vi "Write Shield Count.vi"(7 "function":enum16{"Add", "Subtract"}(ring), 8 "error in (no error)":errorcluster, 11 "Shield in":refnum<class "Shield.lvclass">) -> (0 "error out":errorcluster, 3 "Shield out":refnum<class "Shield.lvclass">)   [LabVIEW 2021, in "Shield.lvclass"]
uses:
  Shield.lvclass
  Shield.lvclass/Shield.ctl
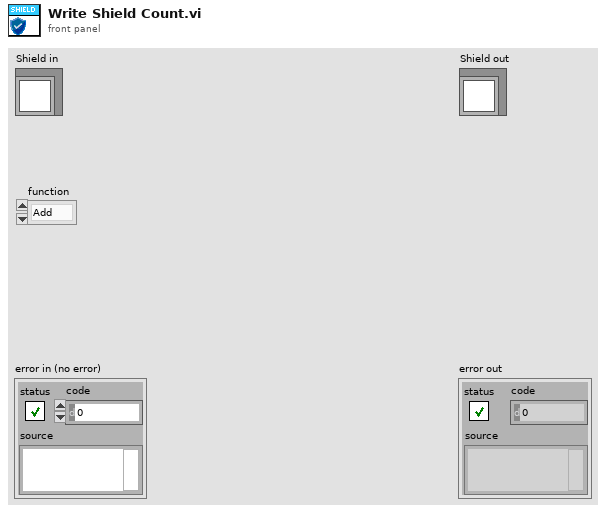
[diagram p1: front panel]
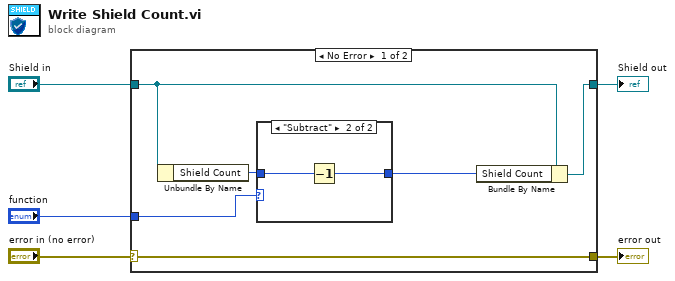
[diagram p0: block diagram]
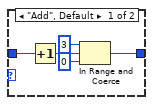
[diagram p2: hidden frame]
diagram:
  n1 = case shown="No Error" "error in (no error)" {
    selector: "error in (no error)" -> [w11 w19]
    tunnel: [w11 w19] -> w4
    tunnel: [w10 w20] -> w2
    tunnel: "Shield in" -> [w7 w20]
    tunnel: "function" -> [w9 _]
    frame No Error {
      n2 = Unbundle By Name(w7) -> ("Shield Count"=w6:u8)
      n3 = case shown="\"Subtract\"" w9 {
        tunnel: w6 -> [w16 w18]
        tunnel: [w14 w17] -> w8
        frame "Add", Default {
          n4 = Increment(x=w16) -> (x+1=w15:u8)
          n5 = In Range and Coerce(upper limit=u8 3, x=w15, lower limit=u8 0) -> (coerced(x)=w14:u8)  [unwired: 1 out]
        }
        frame "Subtract" {
          n6 = Decrement(x=w18) -> (x-1=w17:u8)
        }
      }
      n7 = Bundle By Name(cluster=w7, "Shield Count"=w8) -> (w10:refnum<class "Shield.lvclass">)
    }
    frame Error {
    }
  }
  "error out" <- w4
  "Shield out" <- w2
